vi "test_app.vi"() -> (3 "Waveform Graph":waveform(dbl)(graph))   [LabVIEW 2015]
uses:
  Model/Waveforms/PeriodicWave/PeriodicWave.lvclass
  Typedefs/Iterations.ctl
  Model/Waveforms/ChirpWave/ChirpWave.lvclass
  Typedefs/ChirpWaveInput.ctl
  Model/Waveforms/GuassianNoiseWave/GuassianNoiseWave.lvclass
  Typedefs/GuassianNoiseWaveInput.ctl
  Typedefs/FAMTTypedefs.lvlib
panel:
  in  "Waveforms":T1(ring)
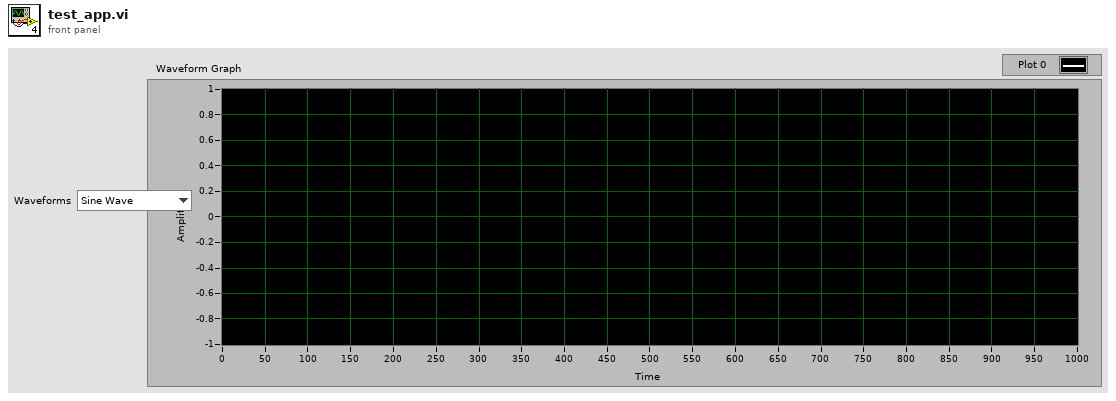
[diagram p1: front panel]
types:
  T1 = enum16{"Sine Wave", "Triangle Wave", "Square Wave", "Sawtooth Wave", "Chirp Wave", "Gaussian Wave"}
  T2 = typedef "FAMTTypedefs.lvlib/Iterations.ctl" = i32
  T3 = cluster{"Offset":dbl, "Frequency":dbl, "Amplitude":dbl, "Phase":dbl, "Duty Cycle":dbl, "Number of Iterations":T2}
  T4 = typedef "FAMTTypedefs.lvlib/ChirpWaveInput.ctl" = cluster{"Amplitude":dbl, "Frequency 1":dbl, "Frequency 2":dbl, "Samples":i32}
  T5 = typedef "FAMTTypedefs.lvlib/GuassianNoiseWaveInput.ctl" = cluster{"Seed":i32, "Standard Deviation":dbl}
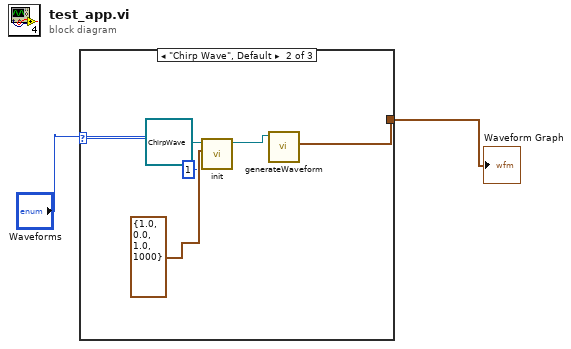
[diagram p0: block diagram]
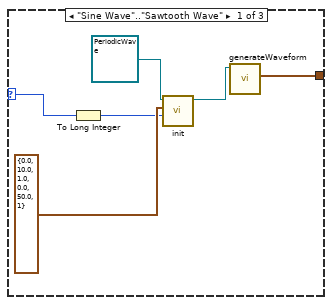
[diagram p2: hidden frame]
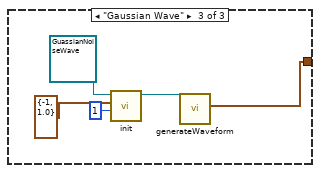
[diagram p3: hidden frame]
diagram:
  n1 = case shown="\"Chirp Wave\", Default" "Waveforms" {
    selector: "Waveforms" -> [w3 _ _]
    tunnel: [w5 w12 w14] -> w2
    frame "Sine Wave".."Sawtooth Wave" {
      n2 = To Long Integer(number=w3) -> (32bit integer=w4:i32)
      n3 = call "init.vi"("Waveforms"=w4, "Inputs to Periodic Wave"=T3 {"Offset"=0.0, "Frequency"=10.0, "Amplitude"=1.0, "Phase"=0.0, "Duty Cycle"=50.0, "Number of Iterations"=1}, "PeriodicWave in"=refnum<class "PeriodicWave.lvclass"> refnum ("PeriodicWave.lvclass")) -> ("PeriodicWave out"=w6:refnum<class "PeriodicWave.lvclass">)  [unwired: 7 in, 1 out]
      n4 = call-dynamic "generateWaveform.vi"("PeriodicWave in"=w6) -> ("signal out"=w5:waveform(dbl))  [unwired: 8 in, 2 out]
    }
    frame "Chirp Wave", Default {
      n5 = call "init.vi"("Number of Iterations"=T2 1, "Input to Chirp Wave"=T4 {"Amplitude"=1.0, "Frequency 1"=0.0, "Frequency 2"=1.0, "Samples"=1000}, "ChirpWave in"=refnum<class "ChirpWave.lvclass"> refnum) -> ("ChirpWave out"=w11:refnum<class "ChirpWave.lvclass">)  [unwired: 7 in, 1 out]
      n6 = call-dynamic "generateWaveform.vi"("ChirpWave in"=w11) -> ("signal out"=w12:waveform(dbl))  [unwired: 8 in, 2 out]
    }
    frame "Gaussian Wave" {
      n7 = call "init.vi"("Number of Iterations"=T2 1, "Inputs to Guassian Noise Wave"=T5 {"Seed"=-1, "Standard Deviation"=1.0}, "GuassianNoiseWave in"=refnum<class "GuassianNoiseWave.lvclass"> refnum) -> ("GuassianNoiseWave out"=w15:refnum<class "GuassianNoiseWave.lvclass">)  [unwired: 7 in, 1 out]
      n8 = call-dynamic "generateWaveform.vi"("GuassianNoiseWave in"=w15) -> ("signal out"=w14:waveform(dbl))  [unwired: 8 in, 2 out]
    }
  }
  "Waveform Graph" <- w2
